vi "TEST - Get Text Label Decs from VI.vi"(8 "error in (no error)":errorcluster) -> (0 "error out":errorcluster, 2 "pass":bool)   [LabVIEW 2020, in "test_openg_application_control.lvlib"]
uses:
  source/library/Close Generic Object Refnum/Close Generic Object Refnum (Array).vi
  source/library/Close Generic Object Refnum/Close Generic Object Refnum (Scalar VI).vi
  test_openg_application_control.lvlib
  <userlib>/_OpenG.lib/error/error.llb/openg_error.lvlib
  source/library/openg_application_control.lvlib
panel:
  # "DO NOT REMOVE"
  # "Test1"
  # "Test2"
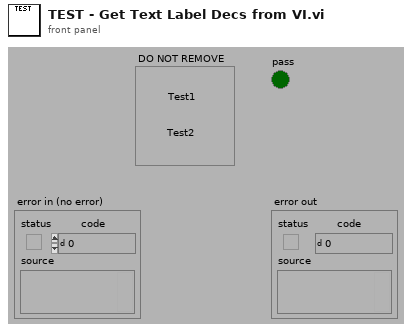
[diagram p1: front panel]
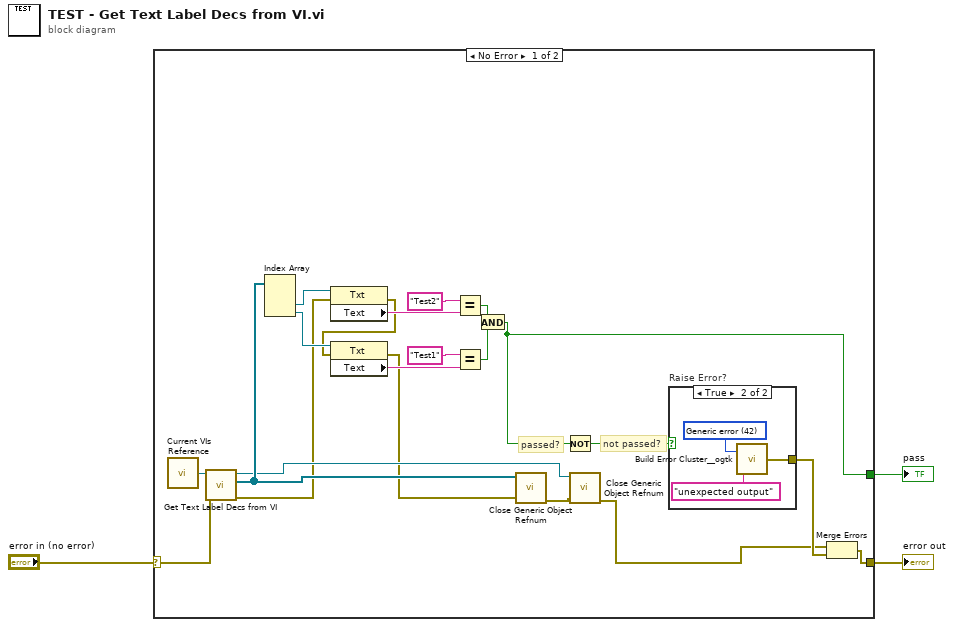
[diagram p0: block diagram]
diagram:
  n1 = case shown="No Error" "error in (no error)" {
    selector: "error in (no error)" -> [w18 w28]
    tunnel: [w7 _] -> w3
    tunnel: [w24 w28] -> w1
    frame No Error {
      # "not passed?"
      # "passed?"
      n2 = call "Current VIs Reference.vi"() -> ("Current VI's reference"=w21:refnum<vi>)  [unwired: 5 in]
      n3 = call "Get Text Label Decs from VI.vi"("error in (no error)"=w18, "VI Refnum"=w21) -> ("error out"=w5:errorcluster, "FP Floating Text Labels"=w20:refnum<vi>[], "dup VI Refnum"=w19:refnum<vi>)  [unwired: 7 in]
      n4 = Index Array(array=w20) -> (element #2=w14:refnum<vi>, element #3=w15:refnum<vi>)  [unwired: 3 in, 1 out]
      n5 = property class="Txt"(reference=w14, error in=w5) -> (error out=w4:errorcluster, "Text"=w13:string)  [unwired: 1 out]
      n6 = property class="Txt"(reference=w15, error in=w4) -> (error out=w6:errorcluster, "Text"=w10:string)  [unwired: 1 out]
      n7 = Equal?(x="Test2", y=w13) -> (x = y?=w9:bool)
      n8 = Equal?(x="Test1", y=w10) -> (x = y?=w8:bool)
      n9 = And(x=w9, y=w8) -> (x .and. y?=w7:bool)
      n10 = call-poly "Close Generic Object Refnum.vi"("error in (no error)"=w6, "Gen Refnum Array"=w20) -> ("error out"=w17:errorcluster)  [unwired: 9 in]
      n11 = Not(x=w7) -> (.not. x?=w22:bool)
      n12 = call-poly "Close Generic Object Refnum.vi"("error in (no error)"=w17, "VI Refnum"=w19) -> ("error out"=w16:errorcluster)  [unwired: 8 in, 1 out]
      n13 = case "Raise Error?" shown="True" w22 {
        tunnel: [_ w25] -> w23
        frame False {
        }
        frame True {
          w26 = 42 items=["No error", "Argument error", "Memory is full", "Out of zone", "End of file", "File already open", "Generic file I/O error", "File not found", "File permission error", "Disk is full", "Duplicate path", "Too many files open", "System feature not enabled", "Resource file not found", "Cannot add resource", "Resource not found", "Image not found", "Image memory error", "Pen does not exist", "Config type invalid", "Config token not found", "Config parse error", "Config memory error", "Bad external code format", "Bad external code offset", "External code not present", "Null window", "Destroy window error", "Null menu", "Print aborted", "Bad print record", "Print driver error", "Windows error during printing", "Memory error during printing", "Print dialog error", "Generic print error", "Invalid device refnum", "Device not found", "Device parameter error", "Device unit error", "Cannot open device", "Device call aborted", "Generic error", "Cancelled by user", "Object ID too low", "Object ID too high", "Object not in heap", "Unknown heap", "Unknown object (invalid DefProc)", "Unknown object (DefProc not in table)", "Message out of range", "Invalid (null) method", "Unknown message", "Manager call not supported", "Bad address", "Network operation in progress", "Network operation timed out", "Connection is busy", "Network attribute not supported", "Network error", "Address in use", "System out of memory", "Connection aborted", "Connection refused", "Not connected", "Already connected", "Connection closed", "Initialization error (interapplication manager)", "Bad occurrence", "Wait on unbound occurrence handler", "Occurrence queue overflow", "Datalog type conflict", "Unused", "Unrecognized type (interapplication manager)", "Memory corrupt", "Failed to make temporary DLL", "Old CIN version", "Drag socket not found", "Failed to load drop-object", "Failed to register OLE object", "Failed to release OLE object", "Format specifier type mismatch", "Unknown format specifier", "Too few format specifiers", "Too many format specifiers", "Scan failed", "Newer CIN version", "Error converting to variant", "Runtime menu error", "Password tampered", "Variant attribute not found", "Incompatible variant data type", "Event data is not available", "Event Store is not present", "Occurrence is not found", "Event Queue is not created", "Event info is not available", "Refnum passed is NULL", "Error retrieving Class GUID", "Error retrieving CoClass GUID", "Error retrieving TypeLib GUID.", "Bad built application magic bytes.", "Specific driver is different from the specific driver associated with the Logical Name.", "There is no session opened to the class driver.", "Max Error", "MAX - Error with config objects", "MAX - Error loading configuration", "MAX - Group not supported"]
          n14 = call <userlib>:"Build Error Cluster__ogtk.vi"("String to Prepend to source (\"\")"="unexpected output" ("String to Prepend to source (\"\")"), "code"=w26) -> ("error out"=w25:errorcluster)
        }
      }
      n15 = Merge Errors(w16, w23) -> (w24:errorcluster)
    }
    frame Error {
    }
  }
  "pass" <- w3
  "error out" <- w1
